vi "Connect.vi"(8 "error in (no error)":errorcluster, 9 "remote port (21)":u16=21, 10 "address":string, 11 "FTP in":refnum<class "FTP.lvclass">) -> (0 "error out":errorcluster, 3 "FTP out":refnum<class "FTP.lvclass">)   [LabVIEW 2020, in "FTP.lvlib" / "FTP.lvclass"]
uses:
  FTP.lvclass
  FTP.lvclass/FTP.ctl
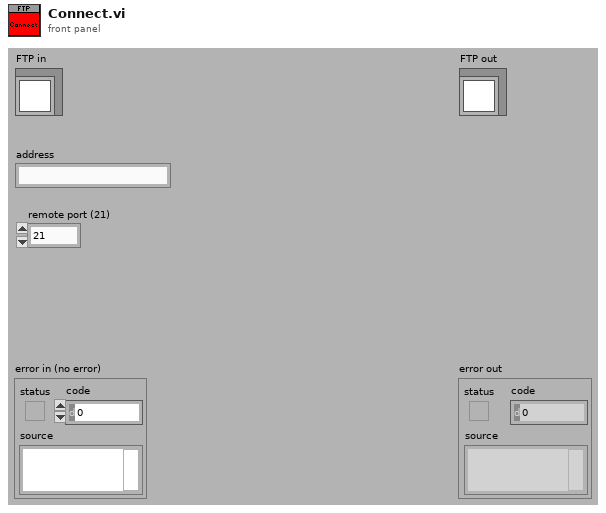
[diagram p1: front panel]
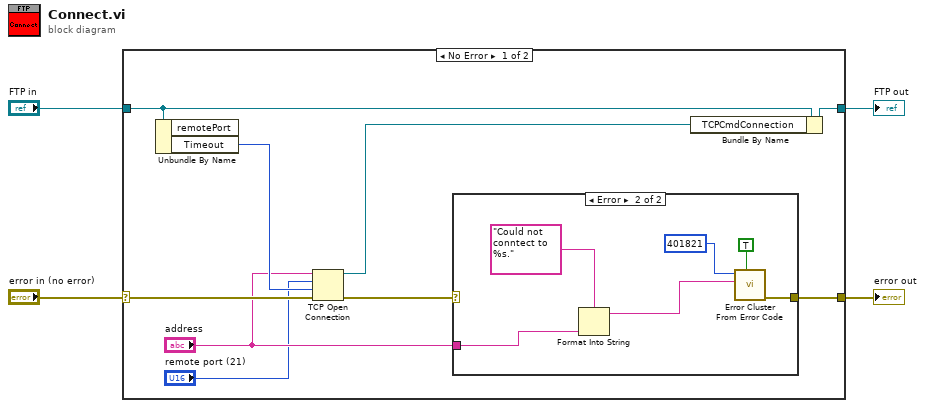
[diagram p0: block diagram]
diagram:
  n1 = case shown="No Error" "error in (no error)" {
    selector: "error in (no error)" -> [w13 w22]
    tunnel: [w8 w22] -> w3
    tunnel: [w10 w21] -> w1
    tunnel: "FTP in" -> [w11 w21]
    frame No Error {
      n2 = Unbundle By Name(w11) -> ("Timeout"=w9:i32)  [unwired: 1 out]
      n3 = TCP Open Connection(address="address", remote port or service name="remote port (21)", timeout ms (60000)=w9, error in (no error)=w13) -> (connection ID=w12:refnum<k5>, error out=w7:errorcluster)  [unwired: 1 in]
      n4 = case shown="Error" w7 {
        selector: w7 -> [w14 _]
        tunnel: [w14 w20] -> w8
        tunnel: "address" -> [_ w17]
        frame No Error {
        }
        frame Error {
          n5 = Format Into String(format string="Could not conntect to %s." ("error message (\"\")"), w17) -> (resulting string=w16:string)  [unwired: 2 in, 1 out]
          n6 = call <vilib>:"Error Cluster From Error Code.vi"("show call chain? (False)"=TRUE, "error message (\"\")"=w16, "error code (0)"=401821) -> ("error out"=w20:errorcluster)  [unwired: 6 in]
        }
      }
      n7 = Bundle By Name(cluster=w11, "TCPCmdConnection"=w12) -> (w10:refnum<class "FTP.lvclass">)
    }
    frame Error {
    }
  }
  "error out" <- w3
  "FTP out" <- w1
